vi "Prueba.vi"   [LabVIEW 2021, in "UDP Comms.lvlib"]
uses:
  UDP Comms.lvlib
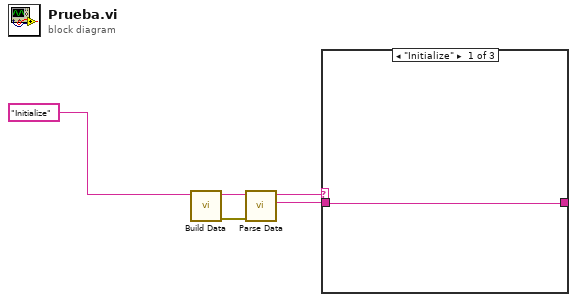
[diagram p0: block diagram]
diagram:
  n1 = call "Build Data.vi"("Command"="Initialize") -> ("error out"=w3:errorcluster, "UDP MSG To be Sent"=w4:string)  [unwired: 9 in]
  n2 = call "Parse Data.vi"("error in (no error)"=w3, 11:w4) -> ("Data"=w1:string, "Command"=w2:string)  [unwired: 7 in, 1 out]
  n3 = case shown="\"Initialize\"" w2 {
    tunnel: w1 -> [w6 w7 w8]
    tunnel: [w6 w7 w8] -> _
    frame "Initialize" {
    }
    frame "Hello World" {
    }
    frame Default {
    }
  }
